vi "Subvi gated pixel clock.vi"(9 "Reset":bool) -> (1 "Gated pixel clock":bool)   [LabVIEW 2017]
uses:
  <vilib>/rvi/Emulation/niFpgaSctlEmulationGetInTimedLoop.vi
  GV Nmax pixel.vi
  GV pixel clock.vi
  GV pixel clock change.vi
  <vilib>/rvi/Emulation/niFpgaProcessEmulError.vi
  Probes/GV DO3.vi
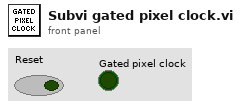
[diagram p1: front panel]
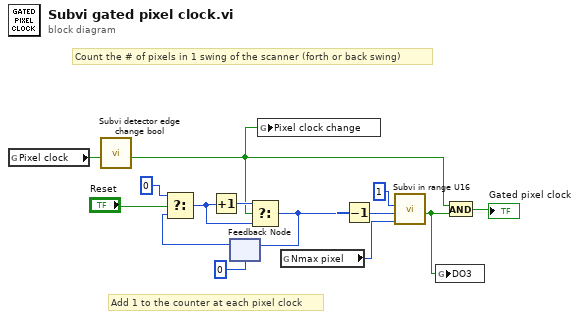
[diagram p0: block diagram]
diagram:
  # "Count the # of pixels in 1 swing of the scanner (forth or back swing)"
  # "Add 1 to the counter at each pixel clock"
  n1 = global read "GV pixel clock.vi" "Pixel clock"() -> (w2:bool)
  n2 = call "Subvi detector edge change bool.vi"("Input"=w2) -> ("Output"=w1:bool)  [unwired: 8 in]
  n3 = feedback #1(u16 0) -> (w11:u16)
  n4 = Select(t=u16 0, s="Reset", f=w11) -> (s? t:f=w12:u16)
  n5 = Increment(x=w12) -> (x+1=w13:u16)
  n6 = Select(t=w13, s=w1, f=w12) -> (s? t:f=w5:u16)
  n7 = feedback-in #1(w5) -> ()
  n8 = global write "GV pixel clock change.vi" "Pixel clock change"(w1) -> ()
  n9 = global read "GV Nmax pixel.vi" "Nmax pixel"() -> (w6:u16)
  n10 = Decrement(x=w5) -> (x-1=w7:u16)
  n11 = call "Subvi in range U16.vi"("Max"=w6, "Input"=w7, "Min"=u16 1) -> ("In range"=w4:bool)  [unwired: 8 in]
  n12 = global write "GV DO3.vi" "DO3"(w4) -> ()
  n13 = And(x=w1, y=w4) -> (x .and. y?=→"Gated pixel clock":bool)
